vi "To XML - With Class - Returns XML Entities.vi"() -> ()   [LabVIEW 2017, in "Cobertura.Tests.lvlib" / "Package.lvlib"]
uses:
  Package.lvlib
  <vilib>/xml/Close Reference(Node).vi
  Cobertura/Package/Package.lvclass
  <vilib>/xml/NI_XML.lvlib
  <resource>/objmgr/DOMUserDefRef.rc
  <vilib>/PNR/Transparent Assertions/Transparent Assertions/Transparent Assertions.lvlib
  Cobertura/Class/Class.lvclass
panel:
  out "error out":errorcluster
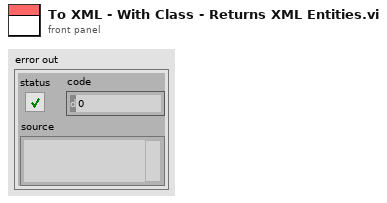
[diagram p1: front panel]
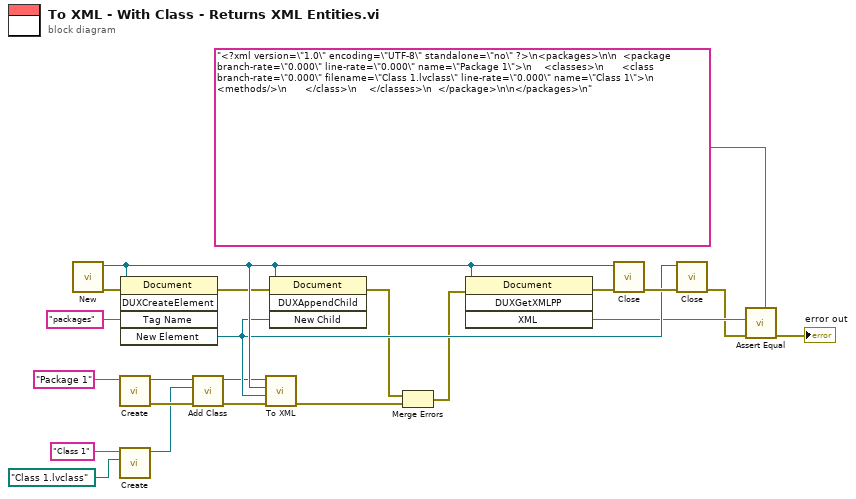
[diagram p0: block diagram]
diagram:
  n1 = call <vilib>:"New.vi"() -> ("error out"=w17:errorcluster, "DOM document out"=w19:refnum<k20>)  [unwired: 8 in]
  n2 = call "Create.vi"("Name"="Package 1") -> ("error out"=w22:errorcluster, "Package"=w3:refnum<class "Package.lvclass">)  [unwired: 9 in]
  n3 = call "Create.vi"("Filename"=path "Class 1.lvclass", "Name"="Class 1") -> ("Class"=w2:refnum<class "Class.lvclass">)  [unwired: 8 in, 1 out]
  n4 = invoke class="Document" method="DUXCreateElement"(reference=w19, error in=w17, "Tag Name"="packages") -> (error out=w18:errorcluster, "New Element"=w15:refnum<k20>)  [unwired: 2 in, 3 out]
  n5 = call "Add Class.vi"("error in (no error)"=w22, "Class"=w2, "Package in"=w3) -> ("error out"=w6:errorcluster, "Package out"=w5:refnum<class "Package.lvclass">)  [unwired: 7 in]
  n6 = call-dynamic "To XML.vi"("error in (no error)"=w6, "Parent"=w15, "Document"=w19, "Package in"=w5) -> ("error out"=w9:errorcluster)  [unwired: 7 in]
  n7 = invoke class="Document" method="DUXAppendChild"(reference=w19, error in=w18, "New Child"=w15) -> (error out=w11:errorcluster)  [unwired: 1 in, 3 out]
  n8 = Merge Errors(w11, w9) -> (w10:errorcluster)
  n9 = invoke class="Document" method="DUXGetXMLPP"(reference=w19, error in=w10) -> (error out=w20:errorcluster, "XML"=w14:string)  [unwired: 2 in, 2 out]
  n10 = call-poly <vilib>:"Close.vi"("error in (no error)"=w20, "node"=w19) -> ("error out"=w16:errorcluster)  [unwired: 7 in]
  n11 = call-poly <vilib>:"Close.vi"("error in (no error)"=w16, "node"=w15) -> ("error out"=w8:errorcluster)  [unwired: 7 in]
  n12 = call <vilib>:"Assert Equal.vi"("Expected"="<?xml version=\"1.0\" encoding=\"UTF-8\" standalone=\"no\" ?>\n<packages>\n\n  <package branch-rate=\"0.000\" line-rate=\"0.000\" name=\"Package 1\">\n    <classes>\n      <class branch-rate=\"0.000\" filename=\"Class 1.lvclass\" line-rate=\"0.000\" name=\"Class 1\">\n        <methods/>\n      </class>\n    </classes>\n  </package>\n\n</packages>\n", "error in (no error)"=w8, "Actual"=w14) -> ("error out"=→"error out":errorcluster)  [unwired: 8 in]
